vi "PH_PSDBWriter.START PSDB THREAD.vi"(0 "VI in":refnum<vi>, 5 "error in (no error)":errorcluster) -> (14 "VI out":refnum<vi>, 19 "error out":errorcluster)   [LabVIEW 2014, in "PH_PSDBWriter.lvlib"]
uses:
  PH_PSDBWriter.lvlib
  CSCore/CSSystem/CSSystemLib/CSSystemLib.lvlib
panel:
  out "created new?":bool
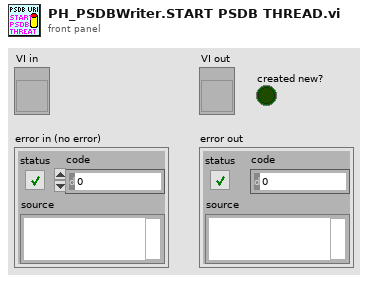
[diagram p1: front panel]
types:
  T1 = typedef "PH_PSDBWriter.lvlib/PH_PSDBWriter.i attribute.ctl" = cluster{"PSDB Status Service ID":i32, "Instance ID":i32, "Shot #":i32, "Subsystem":T2, "Data Status":T3, "Ref PSDB Status":refnum<vi>, "PSDB Error Code":i32, "PSDB Dataset":T4, "PSDB Thread":cluster{"Ref":refnum<vi>, "Q-Ref":refnum<queue>}, "PSDB Credentials":T12}
  T2 = typedef "PH_PSDBWriter.lvlib/PH_PSDBWriter.PHELIX-Subsystems.ctl" = i32
  T3 = typedef "PH_PSDBWriter.lvlib/PH_PSDBWriter.Data Status.ctl" = i16
  T4 = typedef "PH_PSDBWriter.lvlib/PH_PSDBWriter.PSDB Dataset.ctl" = cluster{"Version":i32, "2D data Input":T5[], "Boolean Input":T7[], "Image Input":T8[], "Numeric Input":T10[], "String Input":T11[]}
  T5 = typedef "PH_PSDBWriter.lvlib/PH_PSDBWriter.2D dataset.ctl" = cluster{"name":string, "data":dbl[][], "axis description":T6}
  T6 = typedef "PSDB.lvlib/PSDB_AxisDescription.ctl" = cluster{"x axis label":string, "y axis label":string, "x axis unit":string, "y axis unit":string}
  T7 = typedef "PH_PSDBWriter.lvlib/PH_PSDBWriter.Boolean dataset.ctl" = cluster{"name":string, "data":bool, "unit":string}
  T8 = typedef "PH_PSDBWriter.lvlib/PH_PSDBWriter.Image dataset.ctl" = cluster{"name":string, "data":T9, "unit":string}
  T9 = typedef "IMAQ Image.ctl" = refnum<image>
  T10 = typedef "PH_PSDBWriter.lvlib/PH_PSDBWriter.Numeric dataset.ctl" = cluster{"name":string, "data":dbl, "unit":string}
  T11 = typedef "PH_PSDBWriter.lvlib/PH_PSDBWriter.String dataset.ctl" = cluster{"name":string, "data":string, "unit":string}
  T12 = typedef "PH_Common.lvlib/PH_Connection.PSDB Credentials.ctl" = cluster{"PW":string, "ID":string, "DS":string}
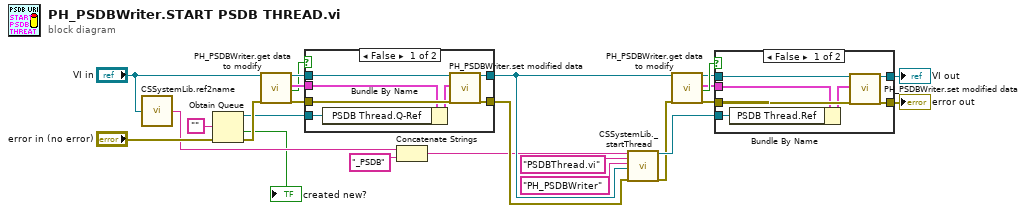
[diagram p0: block diagram]
diagram:
  n1 = call "CSSystemLib.ref2name.vi"("obj refnum"="VI in") -> ("name"=w4:string)
  n2 = Obtain Queue(element data type="", error in (no error)="error in (no error)") -> (queue out=w23:refnum<queue>, created new?=→"created new?":bool, error out=w25:errorcluster)  [unwired: 3 in]
  n3 = call "PH_PSDBWriter.get data to modify.vi"("i ref in"="VI in", "error in (no error)"=w25) -> ("i ref out"=w20:refnum<vi>, "i attribute"=w18:T1, "timed out"=w17:bool, "error out"=w19:errorcluster)  [unwired: 14 in]
  n4 = case shown="False" w17 {
    tunnel: w20 -> [w32 w34]
    tunnel: [w31 w34] -> w22
    tunnel: w19 -> [w30 w33]
    tunnel: [w29 w33] -> w6
    tunnel: w18 -> [w28 _]
    tunnel: w23 -> [w26 _]
    frame False {
      n5 = Bundle By Name(cluster=w28, "PSDB Thread.Q-Ref"=w26) -> (w27:T1)
      n6 = call "PH_PSDBWriter.set modified data.vi"("i ref in"=w32, "i attribute"=w27, "error in (no error)"=w30) -> ("i ref out"=w31:refnum<vi>, "error out"=w29:errorcluster)  [unwired: 15 in]
    }
    frame True {
    }
  }
  n7 = Concatenate Strings(w4, "_PSDB" ("thread name")) -> (w3:string)
  n8 = call "CSSystemLib._startThread.vi"("thread name"=w3, "template name"="PSDBThread.vi", "Class"="PH_PSDBWriter", "object ref"=w22, "error in (no error)"=w6) -> ("thread ref"=w15:refnum<vi>, "error out"=w12:errorcluster)  [unwired: 12 in, 1 out]
  n9 = call "PH_PSDBWriter.get data to modify.vi"("i ref in"=w22, "error in (no error)"=w12) -> ("i ref out"=w9:refnum<vi>, "i attribute"=w14:T1, "timed out"=w16:bool, "error out"=w11:errorcluster)  [unwired: 14 in]
  n10 = case shown="False" w16 {
    tunnel: w9 -> [w41 w43]
    tunnel: [w40 w43] -> w10
    tunnel: w11 -> [w39 w42]
    tunnel: [w38 w42] -> w13
    tunnel: w14 -> [w37 _]
    tunnel: w15 -> [w35 _]
    frame False {
      n11 = Bundle By Name(cluster=w37, "PSDB Thread.Ref"=w35) -> (w36:T1)
      n12 = call "PH_PSDBWriter.set modified data.vi"("i ref in"=w41, "i attribute"=w36, "error in (no error)"=w39) -> ("i ref out"=w40:refnum<vi>, "error out"=w38:errorcluster)  [unwired: 15 in]
    }
    frame True {
    }
  }
  "error out" <- w13
  "VI out" <- w10
